vi "xiCam - AllVIs.vi"   [LabVIEW 2013]
doc: "List of all xiCam VIs used in this library."
uses:
  PRM/PRM/PRM_v2.ctl
types:
  T1 = typedef "PRM_v2.ctl" = enum16{"ACQ_BUFFER_SIZE", "ACQ_FRAME_BURST_COUNT", "ACQ_TIMING_MODE", "ACQ_TRANSPORT_BUFFER_SIZE", "AE_MAX_LIMIT", "AEAG", "AEAG_LEVEL", "API_VERSION", "AG_MAX_LIMIT", "APPLY_CMS", "AUTO_BANDWIDTH_CALCULATION", "AUTO_WB", "AVAILABLE_BANDWIDTH", "AVAILABLE_BANDWIDTH_MAX", "AVAILABLE_BANDWIDTH_MIN", "BPC", "BUFFER_POLICY", "BUFFERS_QUEUE_SIZE", "CC_MATRIX_00", "CC_MATRIX_01", "CC_MATRIX_02", "CC_MATRIX_03", "CC_MATRIX_10", "CC_MATRIX_11", "CC_MATRIX_12", "CC_MATRIX_13", "CC_MATRIX_20", "CC_MATRIX_21", "CC_MATRIX_22", "CC_MATRIX_23", "CC_MATRIX_30", "CC_MATRIX_31", "CC_MATRIX_32", "CC_MATRIX_33", "CHIP_TEMP", "CMS", "COLOR_FILTER_ARRAY", "COOLING", "DEBOUNCE_EN", "DEBOUNCE_POL", "DEBOUNCE_T0", "DEBOUNCE_T1", "DEBUG_LEVEL", "DEFAULT_CC_MATRIX", "DEVICE_INSTANCE_PATH", "DEVICE_MODEL_ID", "DEVICE_NAME", "DEVICE_SN", "DEVICE_TYPE", "DEVICE_USER_ID", "DOWNSAMPLING", "DOWNSAMPLING_MAX", "DOWNSAMPLING_MIN", "DOWNSAMPLING_TYPE", "DRV_VERSION", "EXP_PRIORITY", "EXPOSURE", "EXPOSURE_DIRECT_UPDATE", "EXPOSURE_MAX", "EXPOSURE_MIN", "FFS_FILE_NAME", "FPGA1_VERSION", "FRAMERATE", "FRAMERATE_MAX", "FRAMERATE_MIN", "FREE_FFS_SIZE", "GAIN", "GAIN_DIRECT_UPDATE", "GAIN_MAX", "GAIN_MIN", "GAMMAC", "GAMMAY", "GPI_LEVEL", "GPI_MODE", "GPI_SELECTOR", "GPI_SELECTOR_MAX", "GPI_SELECTOR_MIN", "GPO_MODE", "GPO_SELECTOR", "GPO_SELECTOR_MAX", "GPO_SELECTOR_MIN", "HDR", "HDR_T1", "HDR_T2", "HEIGHT", "HEIGHT_MAX", "HEIGHT_MIN", "HOUSE_TEMP", "IMAGE_DATA_FORMAT", "IMAGE_IS_COLOR", "INPUT_CMS_PROFILE", "IS_COOLED", "IS_DEVICE_EXIST", "KNEEPOINT1", "KNEEPOINT2", "LED_MODE", "LED_SELECTOR", "LED_SELECTOR_MAX", "LED_SELECTOR_MIN", "LIMIT_BANDWIDTH", "LIMIT_BANDWIDTH_MAX", "LIMIT_BANDWIDTH_MIN", "LUT_EN", "LUT_INDEX", "LUT_INDEX_MAX", "LUT_INDEX_MIN", "LUT_VALUE", "LUT_VALUE_MAX", "LUT_VALUE_MIN", "MANUAL_WB", "MCU1_VERSION", "MCU2_VERSION", "OFFSET_X", "OFFSET_X_MAX", "OFFSET_X_MIN", "OFFSET_Y", "OFFSET_Y_MAX", "OFFSET_Y_MIN", "OUTPUT_CMS_PROFILE", "OUTPUT_DATA_BIT_DEPTH", "OUTPUT_DATA_PACKING", "READ_FILE_FFS", "RECENT_FRAME", "SENSOR_DATA_BIT_DEPTH", "SENSOR_MODE", "SENSOR_TAPS", "SHARPNESS", "SHUTTER_TYPE", "TARGET_TEMP", "TRG_DELAY", "TRG_SELECTOR", "TRG_SOFTWARE", "TRG_SOURCE", "USED_FFS_SIZE", "WB_KB", "WB_KG", "WB_KR", "WIDTH", "WIDTH_MAX", "WIDTH_MIN", "WRITE_FILE_FFS", "ACQ_BUFFER_SIZE_UNIT", "ACQ_TRANSPORT_BUFFER_COMMIT", "AEAG_ROI_HEIGHT", "AEAG_ROI_OFFSET_X", "AEAG_ROU_OFFSET_Y", "AEAG_ROI_WIDTH", "API_CONTEXT_LIST", "BINNING_HORIZONTAL", "BINNING_PATTERN", "BINNING_SELECTOR", "BINNING_VERTICAL", "COLUMN_FPN_CORRECTION", "COUNTER_SELECTOR", "COUNTER_VALUE", "DECIMATION_HORIZONTAL", "DECIMATION_PATTERN", "DECIMATION_SELECTOR", "DECIMATION_VERTICAL", "DEVICE_ID", "DEVICE_LOCATION_PATH", "DEVICE_MANIFEST", "DEVICE_RESET", "DEVICE_SENS_SN", "EXPOSURE_BURST_COUNT", "FFS_ACCESS_KEY", "GAIN_SELECTOR", "HW_REVISION", "IMAGE_BLACK_LEVEL", "IMAGE_DATA_BIT_DEPTH", "IMAGE_DATA_FORMAT_RGB32_ALPHA", "IMAGE_PAYLOAD_SIZE", "LENS_APERTURE_VALUE", "LENS_FEATURE", "LENS_FEATURE_SELECTOR", "LENS_FOCAL_LENGTH", "LENS_FOCUS_DISTANCE", "LENS_FOCUS_MOVE", "LENS_FOCUS_MOVEMENT_VALUE", "LENS_MODE", "OUTPUT_DATA_PACKING_TYPE", "SENSOR_CLOCK_FREQ_HZ", "SENSOR_CLOCK_FREQ_INDEX", "SENSOR_FEATURE_SELECTOR", "SENSOR_FEATURE_VALUE", "SENSOR_OUTPUT_CHANNEL_COUNT", "TRANSPORT_PIXEL_FORMAT", "TS_RST_MODE", "TS_RST_SOURCE"}
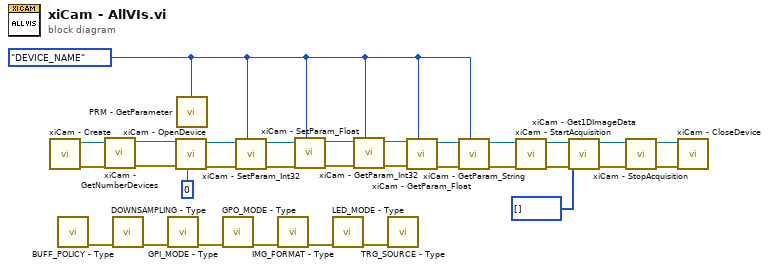
[diagram p0: block diagram]
diagram:
  w12 = PRM_v2."DEVICE_NAME" ("PRM")
  n1 = call "xiCam - Create.vi"() -> ("error out"=w3:errorcluster, "new xiCam"=w5:refnum<k24>)  [unwired: 10 in]
  n2 = call "BUFF_POLICY - Type.vi"() -> ("error out"=w11:errorcluster)  [unwired: 10 in, 1 out]
  n3 = call "xiCam - GetNumberDevices.vi"("error in (no error)"=w3, "xiCam In"=w5) -> ("error out"=w2:errorcluster, "xiCam Out"=w4:refnum<k24>)  [unwired: 7 in, 1 out]
  n4 = call "DOWNSAMPLING - Type.vi"("error in (no error)"=w11) -> ("error out"=w10:errorcluster)  [unwired: 9 in, 1 out]
  n5 = call "GPI_MODE - Type.vi"("error in (no error)"=w10) -> ("error out"=w9:errorcluster)  [unwired: 9 in, 1 out]
  n6 = call "xiCam - OpenDevice.vi"("DevID"=0, "error in (no error)"=w2, "xiCam In"=w4) -> ("error out"=w22:errorcluster, "xiCam Out"=w21:refnum<k24>)  [unwired: 7 in]
  n7 = call "PRM - GetParameter.vi"("PRM"=w12) -> ()  [unwired: 8 in, 3 out]
  n8 = call "GPO_MODE - Type.vi"("error in (no error)"=w9) -> ("error out"=w8:errorcluster)  [unwired: 9 in, 1 out]
  n9 = call "xiCam - SetParam_Int32.vi"("PRM"=w12, "error in (no error)"=w22, "xiCam In"=w21) -> ("error out"=w30:errorcluster, "xiCam Out"=w31:refnum<k24>)  [unwired: 7 in]
  n10 = call "IMG_FORMAT - Type.vi"("error in (no error)"=w8) -> ("error out"=w7:errorcluster)  [unwired: 9 in, 1 out]
  n11 = call "xiCam - SetParam_Float.vi"("PRM"=w12, "error in (no error)"=w30, "xiCam In"=w31) -> ("error out"=w28:errorcluster, "xiCam Out"=w29:refnum<k24>)  [unwired: 7 in]
  n12 = call "LED_MODE - Type.vi"("error in (no error)"=w7) -> ("error out"=w6:errorcluster)  [unwired: 9 in, 1 out]
  n13 = call "xiCam - GetParam_Int32.vi"("PRM"=w12, "error in (no error)"=w28, "xiCam In"=w29) -> ("error out"=w26:errorcluster, "xiCam Out"=w27:refnum<k24>)  [unwired: 6 in, 1 out]
  n14 = call "TRG_SOURCE - Type.vi"("error in (no error)"=w6) -> ()  [unwired: 9 in, 2 out]
  n15 = call "xiCam - GetParam_Float.vi"("PRM"=w12, "error in (no error)"=w26, "xiCam In"=w27) -> ("error out"=w24:errorcluster, "xiCam Out"=w25:refnum<k24>)  [unwired: 6 in, 1 out]
  n16 = call "xiCam - GetParam_String.vi"("PRM"=w12, "error in (no error)"=w24, "xiCam In"=w25) -> ("error out"=w19:errorcluster, "xiCam Out"=w20:refnum<k24>)  [unwired: 6 in, 1 out]
  n17 = call "xiCam - StartAcquisition.vi"("error in (no error)"=w19, "xiCam In"=w20) -> ("error out"=w17:errorcluster, "xiCam Out"=w18:refnum<k24>)  [unwired: 8 in]
  n18 = call "xiCam - Get1DImageData.vi"("error in (no error)"=w17, "1DImageData In"=u8[] [], "xiCam In"=w18) -> ("error out"=w15:errorcluster, "xiCam Out"=w16:refnum<k24>)  [unwired: 5 in, 2 out]
  n19 = call "xiCam - StopAcquisition.vi"("error in (no error)"=w15, "xiCam In"=w16) -> ("error out"=w13:errorcluster, "xiCam Out"=w14:refnum<k24>)  [unwired: 8 in]
  n20 = call "xiCam - CloseDevice.vi"("error in (no error)"=w13, "xiCam In"=w14) -> ()  [unwired: 9 in, 1 out]
